vi "PDC_OpenDevice2.vi"(4 "ConnectMode":i32, 6 "MaxRetryCount":i32, 8 "error in (no error)":errorcluster, 9 "InterfaceCode":u32, 10 "TmpDeviceNo":u32 format="%.0x", 11 "DeviceCode":u32) -> (0 "error out":errorcluster, 1 "DeviceNo":u32, 2 "ErrorCode":u32, 3 "ReturnValue":u32)   [LabVIEW 8.6]
doc: "This VI opens and initializes the specified device.\nThis VI is a function that adds the safe connection mode to PDC_OpenDevice."
uses:
  PDCLIB.dll
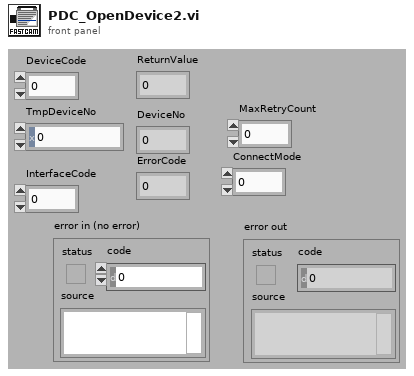
[diagram p1: front panel]
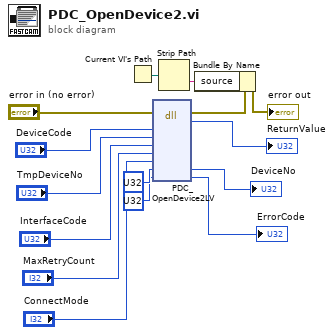
[diagram p0: block diagram]
diagram:
  n1 = Current VI's Path() -> (path=w5:path)
  n2 = dll-call lib="PDCLIB.dll" fn="PDC_OpenDevice2LV"(error in="error in (no error)", "nDeviceCode"="DeviceCode", "nTmpDeviceNo"="TmpDeviceNo", "nInterfaceCode"="InterfaceCode", "nMaxRetryCount"="MaxRetryCount", "nConnectMode"="ConnectMode", "nDeviceNo"=u32 ?, "pErrorCode"=u32 ?) -> (error out=w4:errorcluster, "return type"=→"ReturnValue":u32, "nDeviceNo"=→"DeviceNo":u32, "pErrorCode"=→"ErrorCode":u32)  [unwired: 7 in, 1 out]
  n3 = Strip Path(path=w5) -> (name=w6:string)  [unwired: 1 out]
  n4 = Bundle By Name(cluster=w4, "source"=w6) -> (→"error out":errorcluster)
